vi "Elevator Controller.vi"(8 "error in":errorcluster) -> ()   [LabVIEW 2017]
doc: "This VI executes continuously carrying out the current operation and responding to updates or new operations. It will often contain the timing or control code that is difficult to place directly in TeleOp. This VI generally opens all sensors and motors and isolates the rest of the robot code from knowing how the operations are carried out."
uses:
  <vilib>/Rock Robotics/WPI/Framework/Completion Status.ctl
  Elevator Setpoints.ctl
  Elevator Operations.ctl
  <vilib>/Rock Robotics/WPI/ThirdParty/Phoenix-LabVIEW/Motor Controller/Controls/CTRE_Phoenix_MotorControl_FeedbackDevice.ctl
  <vilib>/Rock Robotics/WPI/ThirdParty/Phoenix-LabVIEW/Motor Controller/Controls/CTRE_Phoenix_MotorControl_LimitSwitchNormal.ctl
  <vilib>/Rock Robotics/WPI/ThirdParty/Phoenix-LabVIEW/Motor Controller/Controls/CTRE_Phoenix_MotorControl_LimitSwitchSource_Local.ctl
  <vilib>/Rock Robotics/WPI/ThirdParty/Phoenix-LabVIEW/Motor Controller/Controls/CTRE_Phoenix_MotorControl_ControlMode.ctl
  <vilib>/Rock Robotics/WPI/ThirdParty/Phoenix-LabVIEW/Motor Controller/Get/CTRE_Phoenix_MotorController_GetSelectedSensorData.vi
  <vilib>/Rock Robotics/Network Tables/NT Write Boolean.vi
  <vilib>/Rock Robotics/WPI/ThirdParty/Phoenix-LabVIEW/Motor Controller/Get/CTRE_Phoenix_MotorController_GetClosedLoopData.vi
panel:
  out "% error":i32(graph)
  out "Position (Raw Sensor Units)":i32
  out "Waveform Chart 2":T1(graph)={"Position (Raw Sensor Units)"=191, "Closed-loop Target"=190}
  in  "Acceleration":i32=200
  in  "Cruise Velocity":i32=2000
  in  "F":dbl=20.0
  in  "P":dbl=22.0
  in  "I":dbl
  in  "D":dbl
  in  "Interactive Values":T2
  out "Current\nCmd":string="Started at  17:26:09.367\n: StayAtHeight,  S 189.7, D 0.000000"
  in  "Buttons":cluster{"Execute Cmd":bool, "Abort Cmd":bool}
  out "Command Timing":cluster{"Start Time (ms)":u32, "Iterations":i32}={"Start Time (ms)"=4054186, "Iterations"=190}
  out "Status":T4=enum."Incomplete"
  # "Tip: It may be helpful to observe inputs and sensor values.\nYou may also want to display tuning or debugging controls."
  # "Interactive Command: You may fill in the settings for a command\nand schedule it with the Execute button. You can observe and abort\nany command while fine tuning the code for the controller."
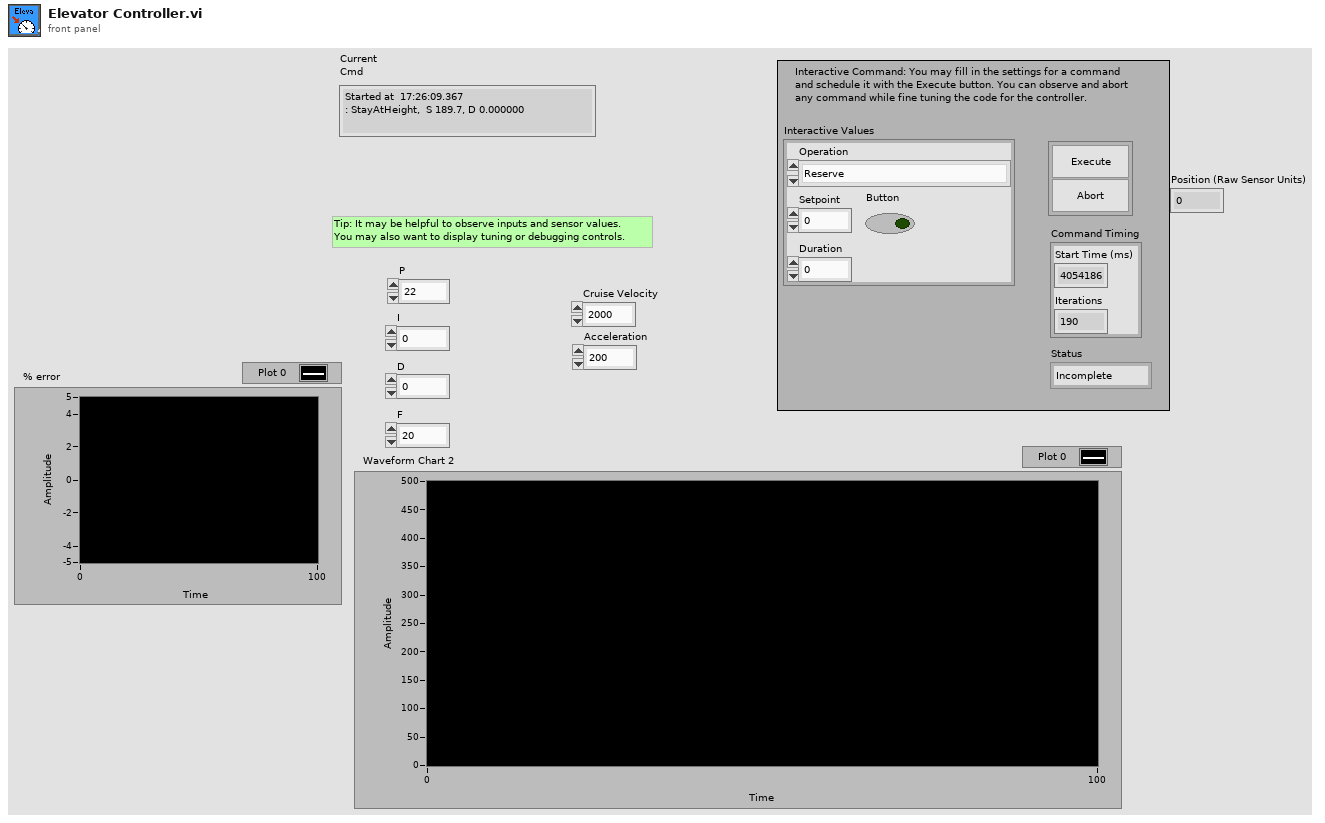
[diagram p1: front panel]
types:
  T1 = cluster{"Position (Raw Sensor Units)":i32, "Closed-loop Target":i32}
  T2 = typedef "Elevator Setpoints.ctl" = cluster{"Operation":T3, "Setpoint":dbl, "Duration":dbl, "Button":bool}
  T3 = typedef "Elevator Operations.ctl" = enum16{"Reserve", "Read Current", "Immediate", "GoToHeight", "StayAtHeight", "LiftForTime"}
  T4 = typedef "Completion Status.ctl" = enum16{"Successful", "Aborted", "Incomplete"}
  T5 = typedef "CTRE_Phoenix_MotorControl_LimitSwitchSource_Local.ctl" = enum16{"Feedback Connector", "Remote Talon SRX", "Remote CANifier", "Deactivated"}
  T6 = typedef "CTRE_Phoenix_MotorControl_LimitSwitchNormal.ctl" = enum16{"Normally Open", "Normally Closed", "Disabled"}
  T7 = typedef "CTRE_Phoenix_MotorControl_FeedbackDevice.ctl" = i8
  T8 = typedef "WPI_MotorControlDeviceRef.ctl" = cluster{"DeviceStatus":errorcluster, "Type":T9, "PWM":cluster{"PWM Channel":T10, "DeadBand":T11}, "CAN":cluster{"Device Number":u8, "SetOutput VI Ref":variant, "GetOutput VI Ref":variant, "Enable VI Ref":variant, "Disable VI Ref":variant, "Data":variant}, "Invert":bool, "DIO PWM":cluster{"PWM \"Enable\" Channel":T10, "DIOChannel":T12, "PWM Rate":dbl}}
  T9 = typedef "WPI_MotorControlType.ctl" = enum16{"PWM", "CAN", "DIO PWM"}
  T10 = typedef "FPGA_DIOPWMChannel.ctl" = enum8{"PWM 0", "PWM 1", "PWM 2", "PWM 3", "PWM 4", "PWM 5", "PWM 6", "PWM 7", "PWM 8", "PWM 9", "PWM MXP 0", "PWM MXP 1", "PWM MXP 2", "PWM MXP 3", "PWM MXP 4", "PWM MXP 5", "PWM MXP 6", "PWM MXP 7", "PWM MXP 8", "PWM MXP 9", "Invalid"}
  T11 = typedef "WPI_PWMDeadband.ctl" = cluster{"Name":string, "maxPositivePwm":i32, "minPositivePwm":i32, "centerPwm":i32, "maxNegativePwm":i32, "minNegativePwm":i32, "angularRange":u16}
  T12 = typedef "FPGA_DIOChannel.ctl" = enum8{"DIO 0", "DIO 1", "DIO 2", "DIO 3", "DIO 4", "DIO 5", "DIO 6", "DIO 7", "DIO 8", "DIO 9", "DIO MXP 0", "DIO MXP 1", "DIO MXP 2", "DIO MXP 3", "DIO MXP 4", "DIO MXP 5", "DIO MXP 6", "DIO MXP 7", "DIO MXP 8", "DIO MXP 9", "DIO MXP 10", "DIO MXP 11", "DIO MXP 12", "DIO MXP 13", "DIO MXP 14", "DIO MXP 15", "SPI Port CS1", "SPI Port CS2", "SPI Port CS3", "SPI Port MISO", "SPI Port MOSI", "Invalid"}
  T13 = typedef "Command Status Info.ctl" = cluster{"Name":string, "Status":T4, "notifier out":T14}
  T14 = typedef "Completion Notifier.ctl" = refnum<notifier>
  T15 = cluster{"Current Command":T2, "Command Timing":cluster{"Start Time (ms)":u32, "Iterations":i32}, "Command Arguments":cluster{"Command Info":T13, "Description":string, "Default Command":T2, "queue out":refnum<queue>, "Subsystem Name":string}}
  T16 = typedef "CTRE_Phoenix_MotorControl_ControlMode.ctl" = u16
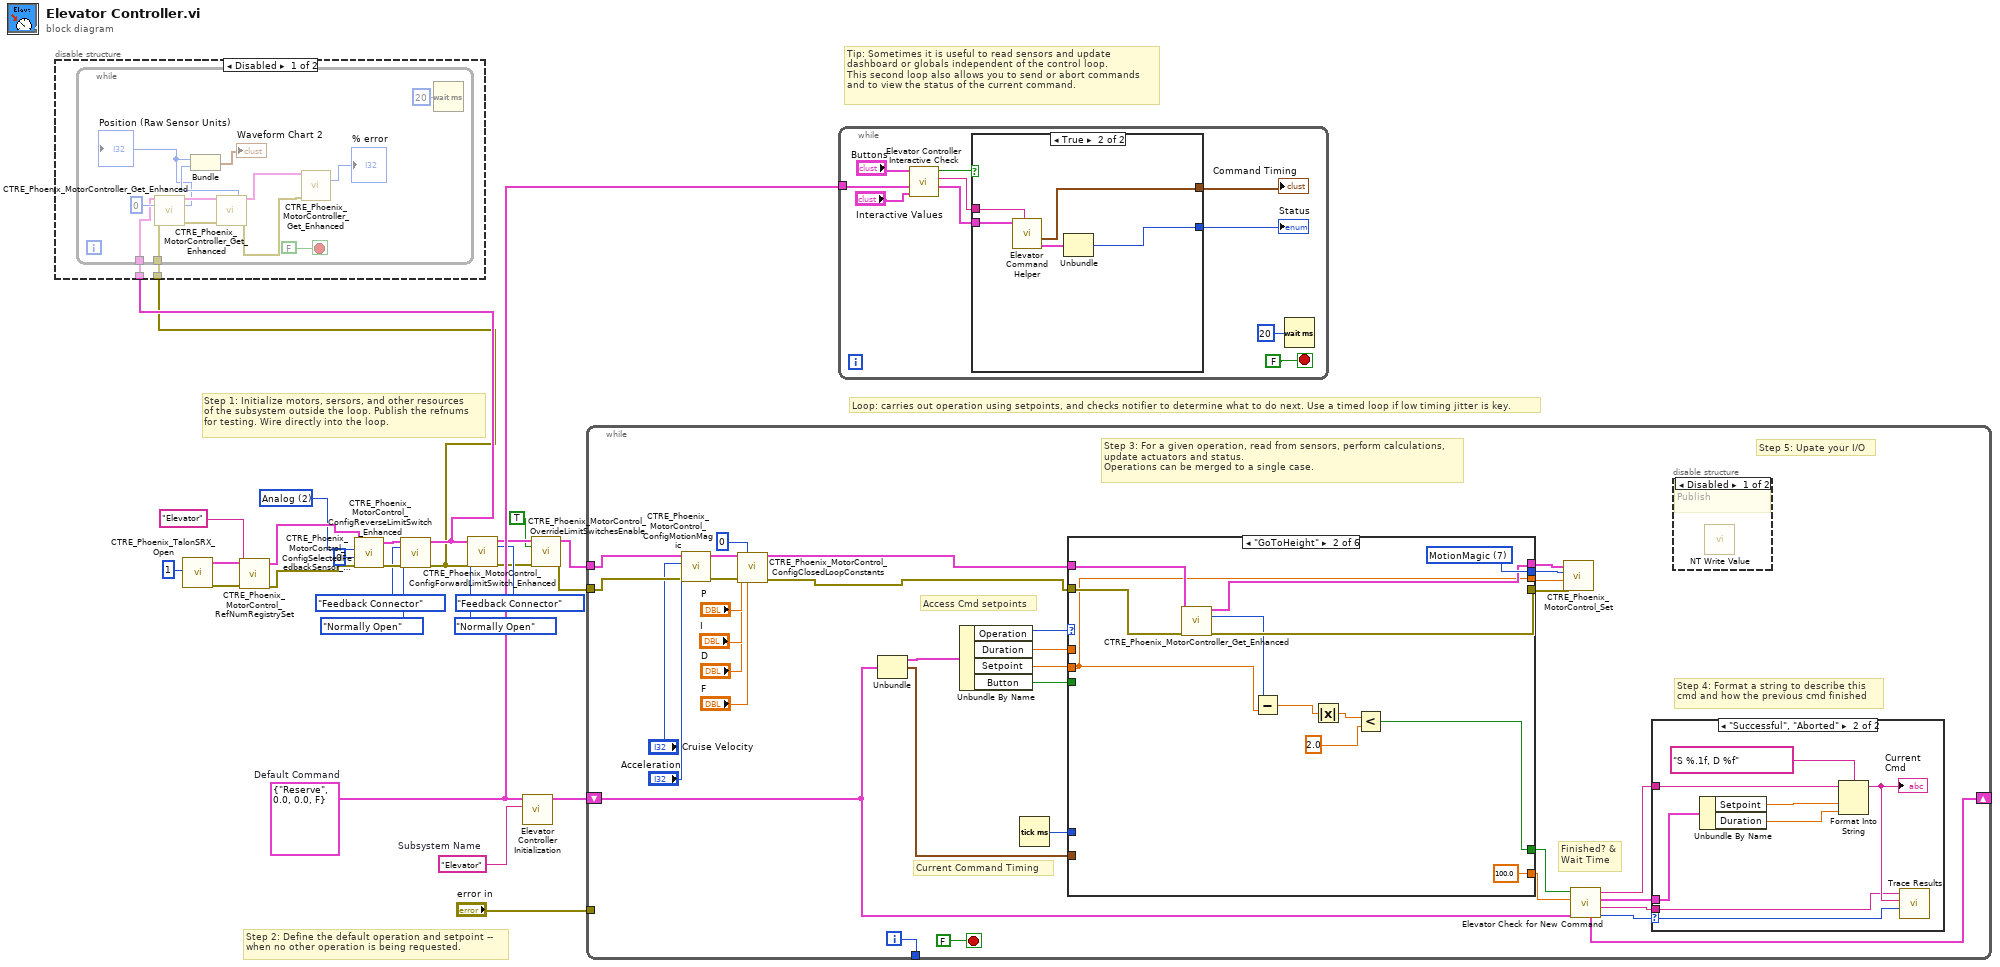
[diagram p0: block diagram]
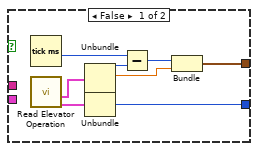
[diagram p3: hidden frame]
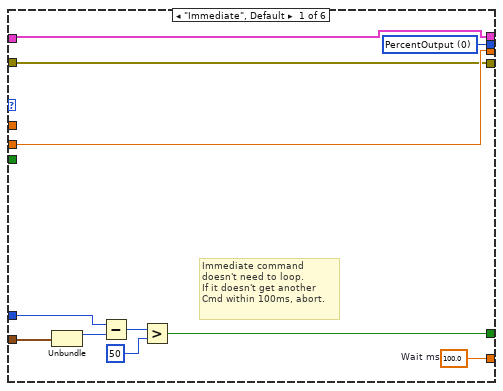
[diagram p6: hidden frame]
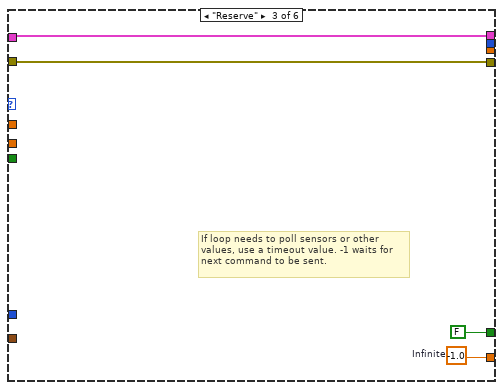
[diagram p7: hidden frame]
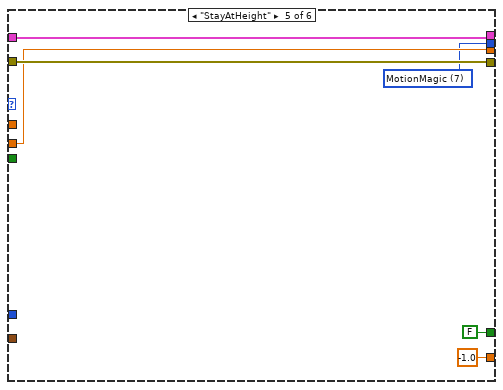
[diagram p9: hidden frame]
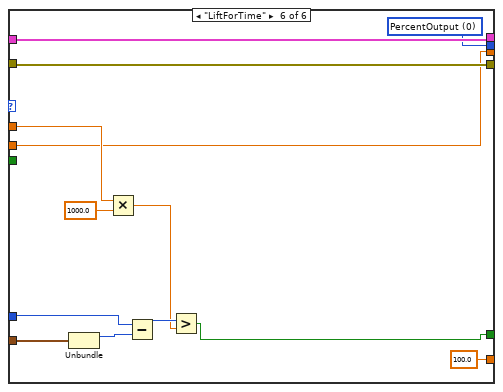
[diagram p10: hidden frame]
diagram:
  w15 = T7 2 items=["None"=-1, "QuadEncoder"=0, "Analog"=2, "Tachometer"=4, "Pulse Width Encoded Position"=8, "Sensor Sum (S0 + S1)"=9, "Sensor Difference (D0 - D1)"=10, "Remote Source 0"=11, "Remote Source 1"=12, "Software Emulated"=15] ("Feedback Device")
  w22 = T2 {"Operation"=enum."Reserve", "Setpoint"=0.0, "Duration"=0.0, "Button"=FALSE}  # Default Command
  w23 = "Elevator"  # Subsystem Name
  # "Tip: Sometimes it is useful to read sensors and update\ndashboard or globals independent of the control loop.\nThis second loop also allows you to send or abort commands\nand to view the status of the current command."
  # "Step 2: Define the default operation and setpoint --\nwhen no other operation is being requested."
  # "Step 1: Initialize motors, sersors, and other resources\nof the subsystem outside the loop. Publish the refnums\nfor testing. Wire directly into the loop."
  # "Loop: carries out operation using setpoints, and checks notifier to determine what to do next. Use a timed loop if low timing jitter is key."
  n1 = call <vilib>:"CTRE_Phoenix_TalonSRX_Open.vi"("Device Number"=u8 1) -> ("error out"=w20:errorcluster, "CAN Talon SRX Ref"=w21:T8)  [unwired: 9 in]
  n2 = call <vilib>:"CTRE_Phoenix_MotorControl_RefNumRegistrySet.vi"("error in (no error)"=w20, "refnum name"="Elevator", "PhoenixMotorControlDevRef"=w21) -> ("error out"=w17:errorcluster, "PhoenixMotorControlDevRef"=w16:T8)  [unwired: 7 in]
  n3 = call <vilib>:"CTRE_Phoenix_MotorControl_ConfigSelectedFeedbackSensor_Enhanced.vi"("error in (no error)"=w17, "pidLoopIdx"=0, "Feedback Device"=w15, "PhoenixMotorControlDevRef"=w16) -> ("error out"=w12:errorcluster, "PhoenixMotorControlDevRef"=w13:T8)  [unwired: 6 in]
  n4 = call <vilib>:"CTRE_Phoenix_MotorControl_ConfigReverseLimitSwitch_Enhanced.vi"("PhoenixMotorControlDevRef"=w13, "Limit Switch Source"=CTRE_Phoenix_MotorControl_LimitSwitchSource_Local."Feedback Connector", "NormallyOpenOrClosed"=CTRE_Phoenix_MotorControl_LimitSwitchNormal."Normally Open", "error in (no error)"=w12) -> ("PhoenixMotorControlDevRef"=w2:T8, "error out"=w1:errorcluster)  [unwired: 10 in]
  n5 = disable-structure shown="Disabled" {
    disable-tunnel: w2 -> [w27 _]
    disable-tunnel: w1 -> [w26 _]
    frame Disabled {
      n6 = while {
        tunnel: w27 -> [w34]
        tunnel: w26 -> [w33]
        stop <- FALSE stop-if-true
        n7 = call-poly <vilib>:"CTRE_Phoenix_MotorController_Get_Enhanced.vi"("PhoenixMotorControlDevRef"=w34, "pidLoopIdx"=u32 0, "error in"=w33) -> ("PhoenixMotorControlDevRef"=w39:T8, "Position (Raw Sensor Units)"=w37:i32, "error out"=w32:errorcluster)  [unwired: 9 in, 1 out]
        "Position (Raw Sensor Units)" <- w37
        n8 = call-poly <vilib>:"CTRE_Phoenix_MotorController_Get_Enhanced.vi"("PhoenixMotorControlDevRef"=w39, "error in"=w32) -> ("Closed-loop Target"=w38:i32, "PhoenixMotorControlDevRef"=w30:T8, "error out"=w29:errorcluster)  [unwired: 8 in, 3 out]
        n9 = Bundle("Position (Raw Sensor Units)"=w37, "Closed-loop Target"=w38) -> (→"Waveform Chart 2":T1)  [unwired: 1 in]
        n10 = call-poly <vilib>:"CTRE_Phoenix_MotorController_Get_Enhanced.vi"("PhoenixMotorControlDevRef"=w30, "error in"=w29) -> ("Closed-loop Error"=→"% error":i32)  [unwired: 8 in, 5 out]
        n11 = Wait (ms)(milliseconds to wait=u32 20) -> ()  [unwired: 1 out]
      }
    }
    frame Enabled {
    }
  }
  n12 = call <vilib>:"CTRE_Phoenix_MotorControl_ConfigForwardLimitSwitch_Enhanced.vi"("PhoenixMotorControlDevRef"=w2, "Limit Switch Source"=CTRE_Phoenix_MotorControl_LimitSwitchSource_Local."Feedback Connector", "NormallyOpenOrClosed"=CTRE_Phoenix_MotorControl_LimitSwitchNormal."Normally Open", "error in (no error)"=w1) -> ("PhoenixMotorControlDevRef"=w7:T8, "error out"=w6:errorcluster)  [unwired: 10 in]
  n13 = call "Elevator Controller Initialization.vi"("Subsystem Name"=w23, "Default Command"=w22) -> ("Current Command"=w24:T15)  [unwired: 9 in]
  n14 = call <vilib>:"CTRE_Phoenix_MotorControl_OverrideLimitSwitchesEnable.vi"("PhoenixMotorControlDevRef"=w7, "Override Limit Switch Enable?"=TRUE, "error in (no error)"=w6) -> ("PhoenixMotorControlDevRef"=w4:T8, "error out"=w3:errorcluster)  [unwired: 11 in]
  n15 = while {
    shift-right: [w67] -> _
    shift-left: w24 -> [w60]
    tunnel: [w73] -> _
    tunnel: "error in" -> [_]
    tunnel: w4 -> [w41]
    tunnel: w3 -> [w47]
    i -> [w73]
    stop <- FALSE stop-if-true
    # "Step 5: Upate your I/O"
    # "Step 4: Format a string to describe this\ncmd and how the previous cmd finished"
    # "Current Command Timing"
    # "Access Cmd setpoints"
    # "Finished? &\nWait Time"
    # "Step 3: For a given operation, read from sensors, perform calculations,\nupdate actuators and status.\nOperations can be merged to a single case."
    n16 = call <vilib>:"CTRE_Phoenix_MotorControl_ConfigMotionMagic.vi"("error in (no error)"=w47, "Acceleration"="Acceleration", "Cruise Velocity"="Cruise Velocity", "PhoenixMotorControlDevRef"=w41) -> ("error out"=w52:errorcluster, "PhoenixMotorControlDevRef"=w51:T8)  [unwired: 6 in]
    n17 = call <vilib>:"CTRE_Phoenix_MotorControl_ConfigClosedLoopConstants.vi"("PhoenixMotorControlDevRef"=w51, "slotIdx"=0, "P"="P", "I"="I", "D"="D", "error in (no error)"=w52, "F"="F") -> ("PhoenixMotorControlDevRef"=w43:T8, "error out"=w42:errorcluster)  [unwired: 7 in]
    n18 = Unbundle(w60) -> ("Current Command"=w72:T2, "Command Timing"=w69:cluster{"Start Time (ms)":u32, "Iterations":i32})  [unwired: 1 out]
    n19 = Unbundle By Name(w72) -> ("Operation"=w71:T3, "Duration"=w70:dbl, "Setpoint"=w68:dbl, "Button"=w45:bool)
    n20 = Tick Count (ms)() -> (millisecond timer value=w59:u32)
    n21 = case shown="\"GoToHeight\"" w71 {
      tunnel: [w93 100.0 ("Infinite") w109 _ -1.0 ("Infinite") 100.0 ("Infinite")] -> w65
      tunnel: [w87 w94 FALSE ("ignore previous (F)") _ FALSE ("ignore previous (F)") w123] -> w66
      tunnel: w69 -> [w89 _ _ _ _ w124]
      tunnel: w70 -> [_ _ _ _ _ w121]
      tunnel: w68 -> [w85 w99 _ _ w115 w118]
      tunnel: w43 -> [w83 w103 w107 w111 w117 w130]
      tunnel: w42 -> [w84 w102 w106 w110 w116 w129]
      tunnel: w59 -> [w88 _ _ _ _ w125]
      tunnel: [w84 w100 w106 w110 w116 w129] -> w58
      tunnel: [w83 w101 w107 w111 w117 w130] -> w57
      tunnel: [w85 w99 _ _ w115 w118] -> w56
      tunnel: [w86 w105 _ _ w113 w128] -> w46
      tunnel: w45 -> [_ _ _ _ _ _]
      frame "Immediate", Default {
        w86 = T16 0 items=["PercentOutput"=0, "Position"=1, "Velocity"=2, "Current"=3, "Follower"=5, "MotionProfile"=6, "MotionMagic"=7, "MotionMagicArc"=8, "MotionProfileArc"=10, "Disabled"=15] ("Control Mode")
        w93 = 100.0  # Wait ms
        # "Immediate command\ndoesn't need to loop.\nIf it doesn't get another\nCmd within 100ms, abort."
        n22 = Unbundle(w89) -> ("Start Time (ms)"=w92:u32)  [unwired: 1 out]
        n23 = Subtract(x=w88, y=w92) -> (x-y=w91:u32)
        n24 = Greater?(x=w91, y=u8 50 ("Left Motor")) -> (0:w87:bool)
      }
      frame "GoToHeight" {
        w105 = T16 7 items=["PercentOutput"=0, "Position"=1, "Velocity"=2, "Current"=3, "Follower"=5, "MotionProfile"=6, "MotionMagic"=7, "MotionMagicArc"=8, "MotionProfileArc"=10, "Disabled"=15] ("Control Mode")
        n25 = call-poly <vilib>:"CTRE_Phoenix_MotorController_Get_Enhanced.vi"("PhoenixMotorControlDevRef"=w103, "error in"=w102) -> ("PhoenixMotorControlDevRef"=w101:T8, "Position (Raw Sensor Units)"=w98:i32, "error out"=w100:errorcluster)  [unwired: 10 in, 1 out]
        n26 = Subtract(x=w98, y=w99) -> (x-y=w97:dbl)
        n27 = Absolute Value(x=w97) -> (abs(x)=w96:dbl)
        n28 = Less?(x=w96, y=2.0) -> (x < y?=w94:bool)
      }
      frame "Reserve" {
        w109 = -1.0  # Infinite
        # "If loop needs to poll sensors or other\nvalues, use a timeout value. -1 waits for\nnext command to be sent."
      }
      frame "Read Current" {
      }
      frame "StayAtHeight" {
        w113 = T16 7 items=["PercentOutput"=0, "Position"=1, "Velocity"=2, "Current"=3, "Follower"=5, "MotionProfile"=6, "MotionMagic"=7, "MotionMagicArc"=8, "MotionProfileArc"=10, "Disabled"=15] ("Control Mode")
      }
      frame "LiftForTime" {
        w128 = T16 0 items=["PercentOutput"=0, "Position"=1, "Velocity"=2, "Current"=3, "Follower"=5, "MotionProfile"=6, "MotionMagic"=7, "MotionMagicArc"=8, "MotionProfileArc"=10, "Disabled"=15] ("Control Mode")
        n29 = Unbundle(w124) -> ("Start Time (ms)"=w126:u32)  [unwired: 1 out]
        n30 = Multiply(x=w121, y=1000.0) -> (x*y=w120:dbl)
        n31 = Subtract(x=w125, y=w126) -> (x-y=w127:u32)
        n32 = Greater?(x=w127, y=w120) -> (0:w123:bool)
      }
    }
    n33 = call <vilib>:"CTRE_Phoenix_MotorControl_Set.vi"("error in (no error)"=w58, "Output"=w56, "Control Mode"=w46, "PhoenixMotorControlDevRef"=w57) -> ()  [unwired: 6 in, 2 out]
    n34 = call "Elevator Check for New Command.vi"("Current Command"=w60, "Wait time (ms)"=w65, "Finished?"=w66) -> ("Completion"=w61:T4, "Subsystem Name"=w62:string, "Current Command"=w63:T2, "Initial Trace String"=w64:string, "NextCommand"=w67:T15)  [unwired: 4 in]
    n35 = case shown="\"Successful\", \"Aborted\"" w61 {
      selector: w61 -> [_ w82]
      tunnel: w64 -> [_ w78]
      tunnel: w63 -> [_ w79]
      tunnel: w62 -> [_ w75]
      frame "Incomplete", Default {
        # "Continuing current command"
      }
      frame "Successful", "Aborted" {
        # "Report and setup for next command"
        n36 = Unbundle By Name(w79) -> ("Setpoint"=w81:dbl, "Duration"=w76:dbl)
        n37 = Format Into String(format string="S %.1f, D %f", initial string=w78, w81, w76) -> (resulting string=w77:string)  [unwired: 1 in, 1 out]
        "Current\nCmd" <- w77
        n38 = call <vilib>:"Trace Results.vi"("Status of previous command"=w82, "Description"=w77, "Subsystem"=w75) -> ()  [unwired: 9 in]
      }
    }
    n39 = disable-structure shown="Disabled" {
      frame Disabled {
        # "Publish"
        n40 = call-poly <vilib>:"NT Write Value.vi"() -> ()  [unwired: 11 in, 1 out]
      }
      frame Enabled {
      }
    }
  }
  n41 = while {
    tunnel: w22 -> [w137]
    stop <- FALSE stop-if-true
    n42 = call "Elevator Controller Interactive Check.vi"("Interactive Command in"="Interactive Values", "Default Command"=w137, "Buttons"="Buttons") -> ("Interactive Command out"=w134:T2, "Trace String"=w135:string, "Schedule"=w136:bool)  [unwired: 6 in]
    n43 = case shown="True" w136 {
      tunnel: [w148 w153] -> w133
      tunnel: w134 -> [_ w151]
      tunnel: [w144 w149] -> w132
      tunnel: w135 -> [_ w152]
      frame False {
        n44 = Tick Count (ms)() -> (millisecond timer value=w143:u32)
        n45 = call "Read Elevator Operation.vi"() -> ("Command Info"=w141:T13, "SubSystem Data"=w142:T2)  [unwired: 9 in, 1 out]
        n46 = Unbundle(w142) -> ("Operation"=w147:T3, "Setpoint"=w145:dbl)  [unwired: 2 out]
        n47 = Unbundle(w141) -> ("Status"=w148:T4)  [unwired: 2 out]
        n48 = Subtract(x=w143, y=w147) -> (x-y=w146:u32)
        n49 = Bundle(w146, "Setpoint"=w145) -> (w144:cluster{u32, "Setpoint":dbl})  [unwired: 1 in]
      }
      frame True {
        n50 = call "Elevator Command Helper.vi"("Description"=w152, "SubSystem Data"=w151) -> ("Command Info Out"=w150:T13, "Command Timing"=w149:cluster{"Start Time (ms)":u32, "Iterations":i32})  [unwired: 7 in, 1 out]
        n51 = Unbundle(w150) -> ("Status"=w153:T4)  [unwired: 2 out]
      }
    }
    "Status" <- w133
    "Command Timing" <- w132
    n52 = Wait (ms)(milliseconds to wait=u32 20) -> ()  [unwired: 1 out]
  }
